vi "Mode Stop Pump.vi"(0 "reference in":refnum<class "Stand.lvclass">, 11 "error in (no error)":errorcluster) -> (4 "reference out":refnum<class "Stand.lvclass">, 6 "Done":bool, 15 "error out":errorcluster)   [LabVIEW 2019, in "Stand.lvclass"]
uses:
  Stand.lvclass
  D:/GIT H4000/H4000/src/Device_class/Device.lvclass
  Device_class/Device.lvclass/Device.ctl
  Stand.lvclass/Stand.ctl
  TypeDef/Active Motor.ctl
  TypeDef/Motor N.ctl
  FPGA_API_class/FPGA API.lvclass
  Device_class/Device.lvclass
  PM_Group_class/PM_Group.lvclass
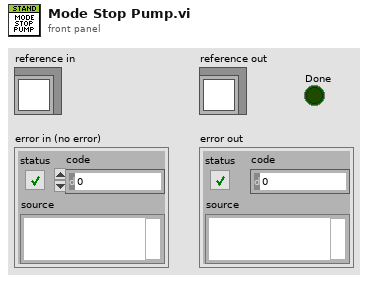
[diagram p1: front panel]
types:
  T1 = typedef "Active Motor.ctl" = cluster{"Active":bool, "MotorN":T2}
  T2 = typedef "Motor N.ctl" = enum16{"M12", "M21", "M24"}
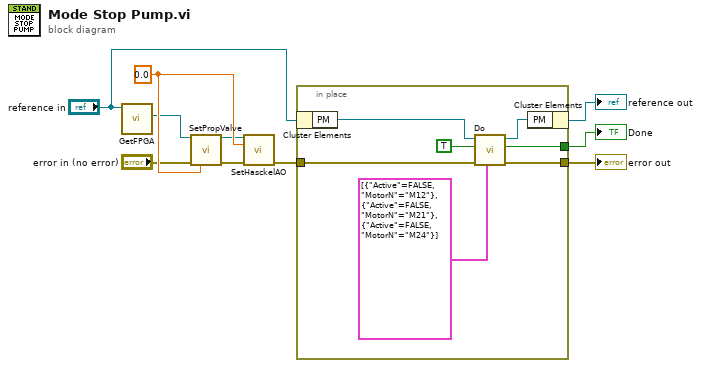
[diagram p0: block diagram]
diagram:
  w10 = 0.0 ("AO 1")
  n1 = call "GetFPGA.vi"("Device in"="reference in") -> ("FPGA API.lvclass"=w6:refnum<class "FPGA API.lvclass">)  [unwired: 10 in]
  n2 = call-dynamic "SetPropValve.vi"("FPGA API in"=w6, "error in (no error)"="error in (no error)", "AO 1"=w10) -> ("FPGA API out"=w7:refnum<class "FPGA API.lvclass">, "error out"=w8:errorcluster)  [unwired: 11 in]
  n3 = call-dynamic "SetHasckelAO.vi"("FPGA API in"=w7, "Haskel in"=w10, "error in (no error)"=w8) -> ("error out"=w9:errorcluster)  [unwired: 11 in, 1 out]
  n4 = in-place {
    in-place-border: w9 -> [w16]
    in-place-border: [w14] -> w4
    in-place-border: [w11] -> w1
    n5 = in-place-cluster #1("reference in") -> ("PM"=w17:refnum<class "PM_Group.lvclass">)
    n6 = call "Do.vi"("Data"=T1[] [{"Active"=FALSE, "MotorN"=enum."M12"}, {"Active"=FALSE, "MotorN"=enum."M21"}, {"Active"=FALSE, "MotorN"=enum."M24"}] ("Array"), "error in (no error)"=w16, "Do"=TRUE, "PM_Group in"=w17) -> ("error out"=w14:errorcluster, "Done"=w11:bool, "PM_Group out"=w15:refnum<class "PM_Group.lvclass">)  [unwired: 5 in]
    n7 = in-place-cluster #1("PM"=w15) -> (→"reference out":refnum<class "Stand.lvclass">)
  }
  "error out" <- w4
  "Done" <- w1
